vi "util_LaserCalibration-VoP.vi"(0 "Vo":dbl[](array[numeric]), 1 "Laser":enum16{"473nm", "532nm"}(ring)) -> (7 "P (mW)":dbl[](array[numeric]))   [LabVIEW 2012]
uses:
  <vilib>/Analysis/NI_AALPro.lvlib
panel:
  out "Power (mW) vs. Voltage":cluster{dbl[], dbl[]}[](graph)
  out "intercept":dbl
  out "slope":dbl
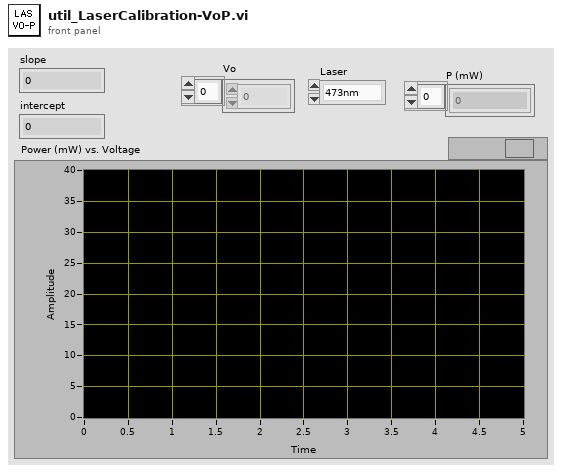
[diagram p1: front panel]
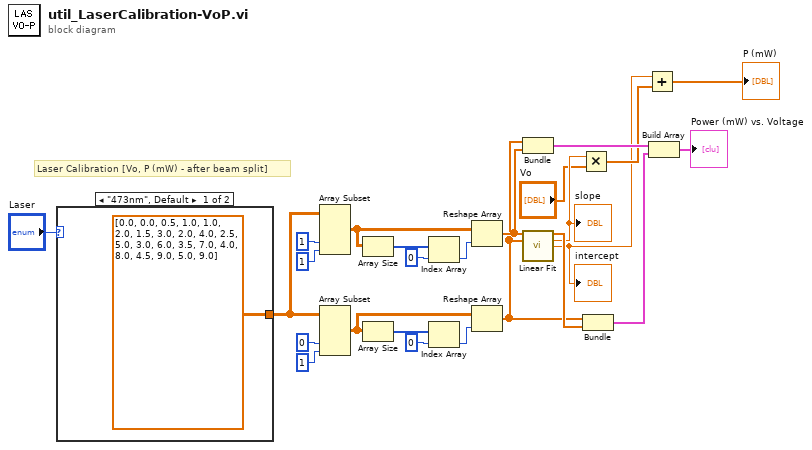
[diagram p0: block diagram]
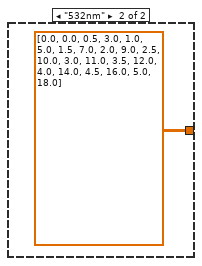
[diagram p2: hidden frame]
diagram:
  # "Laser Calibration [Vo, P (mW) - after beam split]"
  n1 = case shown="\"473nm\", Default" "Laser" {
    tunnel: [dbl[][] [[0.0, 0.0], [0.5, 1.0], [1.0, 2.0], [1.5, 3.0], [2.0, 4.0], [2.5, 5.0], [3.0, 6.0], [3.5, 7.0], [4.0, 8.0], [4.5, 9.0], [5.0, 9.0]] dbl[][] [[0.0, 0.0], [0.5, 3.0], [1.0, 5.0], [1.5, 7.0], [2.0, 9.0], [2.5, 10.0], [3.0, 11.0], [3.5, 12.0], [4.0, 14.0], [4.5, 16.0], [5.0, 18.0]]] -> w13
    frame "473nm", Default {
    }
    frame "532nm" {
    }
  }
  n2 = Array Subset(array=w13, index (col)=1 ("index"), length (col)=1 ("length")) -> (w20:dbl[][])  [unwired: 2 in]
  n3 = Array Subset(array=w13, index (col)=0 ("index"), length (col)=1 ("length")) -> (w14:dbl[][])  [unwired: 2 in]
  n4 = Array Size(array=w20) -> (size(s)=w22:i32[])
  n5 = Array Size(array=w14) -> (size(s)=w16:i32[])
  n6 = Index Array(array=w22, index=0) -> (element=w21:i32)
  n7 = Index Array(array=w16, index=0) -> (element=w15:i32)
  n8 = Reshape Array(w20, w21) -> (w10:dbl[])
  n9 = Reshape Array(w14, w15) -> (w7:dbl[])
  n10 = Bundle(w7, w10) -> (w9:cluster{dbl[], dbl[]})  [unwired: 1 in]
  n11 = call <vilib>:"Linear Fit.vi"("Y"=w10, "X"=w7) -> ("Best Linear Fit"=w8:dbl[], "slope"=w6:dbl, "intercept"=w4:dbl)  [unwired: 9 in, 2 out]
  "slope" <- w6
  "intercept" <- w4
  n12 = Multiply(x=w6, y="Vo") -> (x*y=w5:dbl[])
  n13 = Bundle(w7, "Best Linear Fit"=w8) -> (w11:cluster{dbl[], "Best Linear Fit":dbl[]})  [unwired: 1 in]
  n14 = Add(x=w4, y=w5) -> (x+y=→"P (mW)":dbl[])
  n15 = Build Array(w9, w11) -> (→"Power (mW) vs. Voltage":cluster{dbl[], "Best Linear Fit":dbl[]}[])
